vi "Create Gradient Array.vi"(8 "Values to Include":enum16{"Start", "End", "Start and End", "None"}(ring)=enum."Start and End", 9 "Array Length":dbl, 10 "End Value":dbl, 11 "Start Value":dbl) -> (3 "Output Array":dbl[](array[numeric]))   [LabVIEW 2016]
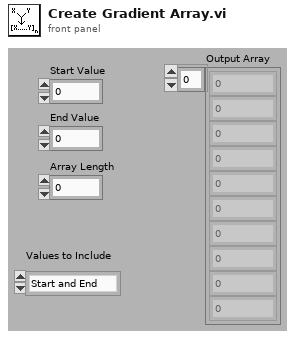
[diagram p1: front panel]
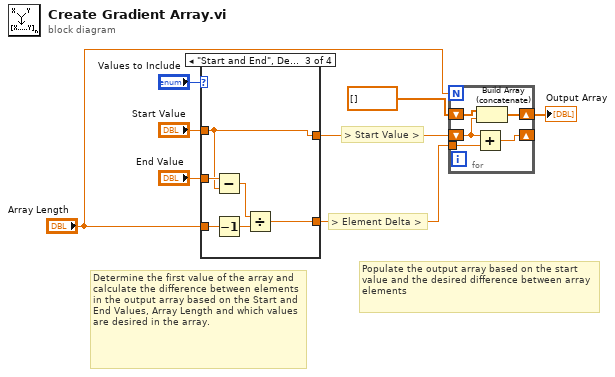
[diagram p0: block diagram]
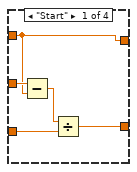
[diagram p2: hidden frame]
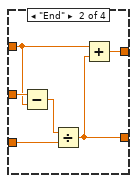
[diagram p3: hidden frame]
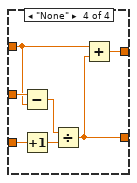
[diagram p4: hidden frame]
diagram:
  # "Populate the output array based on the start value and the desired difference between array elements"
  # "> Element Delta >"
  # "> Start Value >"
  # "Determine the first value of the array and calculate the difference between elements in the output array based on the Start and End Values, Array Length and which values are desired in the array."
  n1 = case shown="\"Start and End\", Default" "Values to Include" {
    tunnel: "End Value" -> [w11 w18 w22 w30]
    tunnel: [w12 w16 w23 w27] -> w7
    tunnel: "Array Length" -> [w10 w17 w21 w29]
    tunnel: "Start Value" -> [w9 w14 w20 w26]
    tunnel: [w9 w15 w20 w28] -> w2
    frame "Start" {
      n2 = Subtract(x=w11, y=w9) -> (x-y=w13:dbl)
      n3 = Divide(x=w13, y=w10) -> (x/y=w12:dbl)
    }
    frame "End" {
      n4 = Subtract(x=w18, y=w14) -> (x-y=w19:dbl)
      n5 = Divide(x=w19, y=w17) -> (x/y=w16:dbl)
      n6 = Add(x=w14, y=w16) -> (x+y=w15:dbl)
    }
    frame "Start and End", Default {
      n7 = Subtract(x=w22, y=w20) -> (x-y=w25:dbl)
      n8 = Decrement(x=w21) -> (x-1=w24:dbl)
      n9 = Divide(x=w25, y=w24) -> (x/y=w23:dbl)
    }
    frame "None" {
      n10 = Subtract(x=w30, y=w26) -> (x-y=w31:dbl)
      n11 = Increment(x=w29) -> (x+1=w32:dbl)
      n12 = Divide(x=w31, y=w32) -> (x/y=w27:dbl)
      n13 = Add(x=w26, y=w27) -> (x+y=w28:dbl)
    }
  }
  n14 = for {
    N: "Array Length" -> [_]
    tunnel: w7 -> [w37]
    shift-right: [w36] -> _
    shift-left: w2 -> [w33]
    shift-right: [w35] -> w5
    shift-left: dbl[] [] -> [w34]
    n15 = Add(x=w33, y=w37) -> (x+y=w36:dbl)
    n16 = Build Array (concatenate)(w34, w33) -> (w35:dbl[])
  }
  "Output Array" <- w5
